vi "Program Sensitivity.vi"(0 "Model in":refnum<class "Model.lvclass">, 11 "error in (no error)":errorcluster) -> (4 "Model out":refnum<class "Model.lvclass">, 15 "error out":errorcluster)   [LabVIEW 2016, in "Model.lvclass"]
uses:
  Model.lvclass
  Model.lvclass/Model.ctl
  Modbus/DesktopModbus/DesktopModbus.lvclass
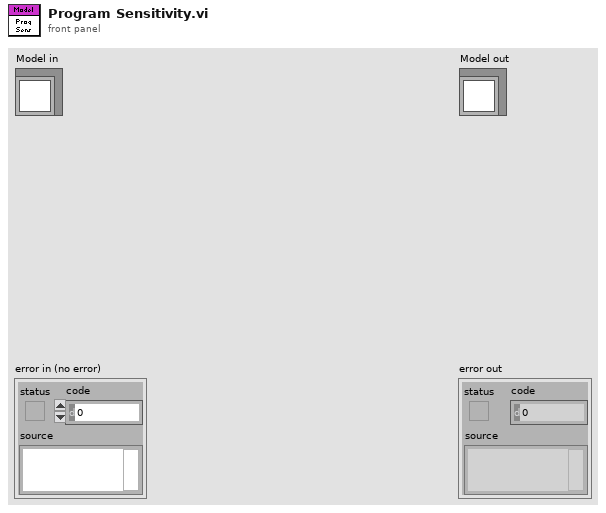
[diagram p1: front panel]
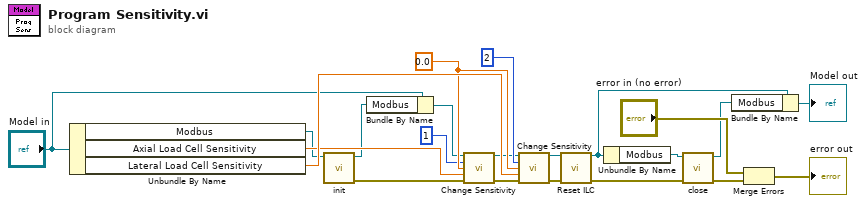
[diagram p0: block diagram]
diagram:
  w20 = sgl 0.0 ("Offset")
  n1 = Unbundle By Name("Model in") -> ("Modbus"=w15:refnum<class "DesktopModbus.lvclass">, "Axial Load Cell Sensitivity"=w17:dbl, "Lateral Load Cell Sensitivity"=w21:dbl)
  n2 = call "init.vi"("DesktopModbus in"=w15) -> ("error out"=w5:errorcluster, "DesktopModbus out"=w11:refnum<class "DesktopModbus.lvclass">)  [unwired: 9 in]
  n3 = Bundle By Name(cluster="Model in", "Modbus"=w11) -> (w6:refnum<class "Model.lvclass">)
  n4 = call "Change Sensitivity.vi"("Model in"=w6, "Channel"=u8 1, "Offset"=w20, "Sensitivity"=w17, "error in (no error)"=w5) -> ("Model out"=w18:refnum<class "Model.lvclass">, "error out"=w22:errorcluster)  [unwired: 9 in]
  n5 = call "Change Sensitivity.vi"("Model in"=w18, "Channel"=u8 2, "Offset"=w20, "Sensitivity"=w21, "error in (no error)"=w22) -> ("Model out"=w4:refnum<class "Model.lvclass">, "error out"=w2:errorcluster)  [unwired: 9 in]
  n6 = call "Reset ILC.vi"("Model in"=w4, "error in (no error)"=w2) -> ("Model out"=w3:refnum<class "Model.lvclass">, "error out"=w1:errorcluster)  [unwired: 12 in]
  n7 = Unbundle By Name(w3) -> ("Modbus"=w10:refnum<class "DesktopModbus.lvclass">)
  n8 = call "close.vi"("error in (no error)"=w1, "DesktopModbus in"=w10) -> ("error out"=w7:errorcluster, "DesktopModbus out"=w9:refnum<class "DesktopModbus.lvclass">)  [unwired: 8 in]
  n9 = Bundle By Name(cluster=w3, "Modbus"=w9) -> (→"Model out":refnum<class "Model.lvclass">)
  n10 = Merge Errors("error in (no error)", w7) -> (→"error out":errorcluster)
